vi "PFE Reserve Cofactor.vi"(7 "tolerance":dbl, 8 "Co-factor Poles":cdb[](array[numeric]), 9 "Poles In":cdb[](array[numeric]), 10 "Multiplicity In":i32[](array[numeric]), 11 "Residues In":cdb[][](array[numeric])) -> (1 "Poles Out":cdb[](array[numeric]), 2 "Multiplicity Out":i32[](array[numeric]), 3 "Residues Out":cdb[][](array[numeric]))   [LabVIEW 2014, in "NI_AALPro.lvlib"]
uses:
  NI_AALPro.lvlib
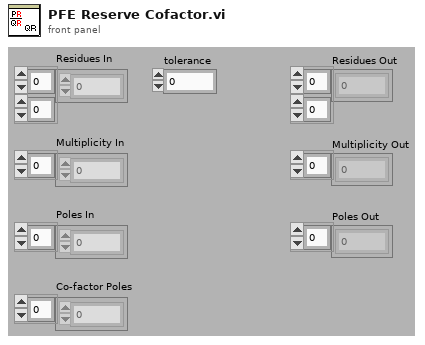
[diagram p1: front panel]
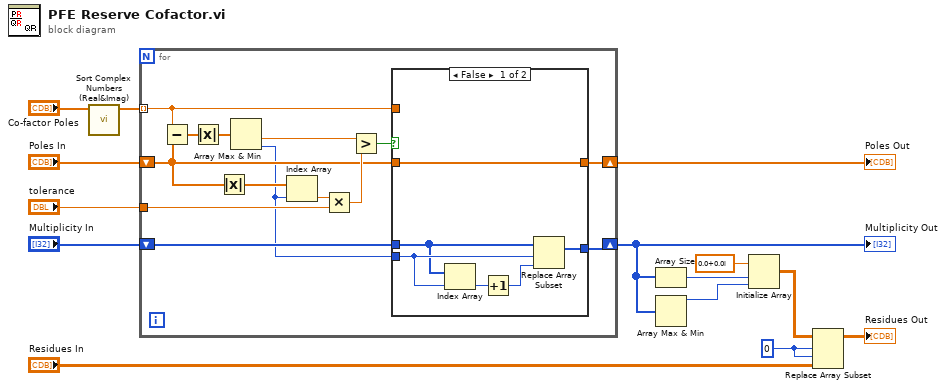
[diagram p0: block diagram]
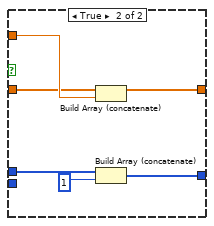
[diagram p2: hidden frame]
diagram:
  w3 = 0 ("index (row)")
  n1 = call "Sort Complex Numbers (Real&Imag).vi"("Complex Numbers"="Co-factor Poles") -> ("Sorted Complex Numbers"=w11:cdb[])  [unwired: 8 in, 2 out]
  n2 = for {
    shift-right: [w18] -> w9
    shift-left: "Poles In" -> [w20]
    shift-right: [w16] -> w8
    shift-left: "Multiplicity In" -> [w17]
    tunnel: "tolerance" -> [w25]
    tunnel: w11 -> [w21] mode=indexing
    n3 = Subtract(x=w21, y=w20) -> (x-y=w28:cdb[])
    n4 = Absolute Value(x=w28) -> (abs(x)=w27:dbl[])
    n5 = Absolute Value(x=w20) -> (abs(x)=w19:dbl[])
    n6 = Array Max & Min(array=w27) -> (min value=w24:dbl, min index (indices)=w15:i32)  [unwired: 2 out]
    n7 = Index Array(array=w19, index=w15) -> (element=w26:dbl)
    n8 = Multiply(x=w26, y=w25) -> (x*y=w23:dbl)
    n9 = Greater?(x=w24, y=w23) -> (0:w22:bool)
    n10 = case shown="False" w22 {
      tunnel: w21 -> [_ w40]
      tunnel: w20 -> [w34 w39]
      tunnel: [w34 w38] -> w18
      tunnel: w17 -> [w32 w37]
      tunnel: [w29 w36] -> w16
      tunnel: w15 -> [w33 _]
      frame False {
        n11 = Index Array(array=w32, index=w33) -> (element=w31:i32)
        n12 = Increment(x=w31) -> (x+1=w30:i32)
        n13 = Replace Array Subset(array=w32, new element=w30, index=w33) -> (w29:i32[])
      }
      frame True {
        n14 = Build Array (concatenate)(w39, w40) -> (w38:cdb[])
        n15 = Build Array (concatenate)(w37, 1) -> (w36:i32[])
      }
    }
  }
  "Poles Out" <- w9
  "Multiplicity Out" <- w8
  n16 = Array Size(array=w8) -> (size(s)=w7:i32)
  n17 = Array Max & Min(array=w8) -> (max value=w6:i32)  [unwired: 3 out]
  n18 = Initialize Array(cdb 0.0+0.0i, w7, w6) -> (w4:cdb[][])
  n19 = Replace Array Subset(array=w4, new element="Residues In", index (row)=w3, index (col)=w3) -> (→"Residues Out":cdb[][])
